vi "Write All Elements Hidden.vi"(8 "error in (no error)":errorcluster, 10 "Config. params. hidden":T1={"Image border size"=1, "Framegrabber board"=0, "Framegrabber buffer"=1, "Camera config file"=path "Support files/camera-config.mcf", "Framegrabber DLL file"=path "C:/CameraVision/Configuration/camera-config.mcf"} {"Framegrabber buffer" min=1; "Framegrabber board" min=0; "Image border size" min=0}, 11 "Config params in":refnum<class "CV-Configuration.lvclass">) -> (0 "error out":errorcluster, 3 "Config params out":refnum<class "CV-Configuration.lvclass">)   [LabVIEW 2013, in "CameraVision.lvlib" / "CV-Configuration.lvclass"]
uses:
  CV-Configuration.lvclass
  Configuration-parameters-advanced.ctl
  CV-Configuration.lvclass/CV-Configuration.ctl
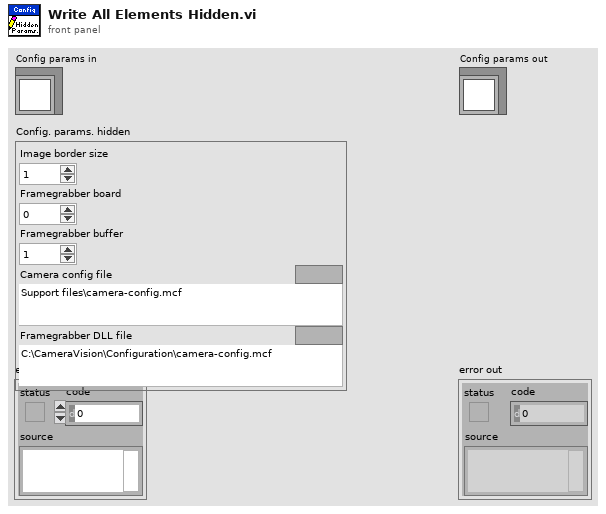
[diagram p1: front panel]
types:
  T1 = typedef "CameraVision.lvlib/CV-Configuration.lvclass/Configuration-parameters-advanced.ctl" = cluster{"Image border size":i32, "Framegrabber board":i32, "Framegrabber buffer":i32, "Camera config file":path, "Framegrabber DLL file":path}
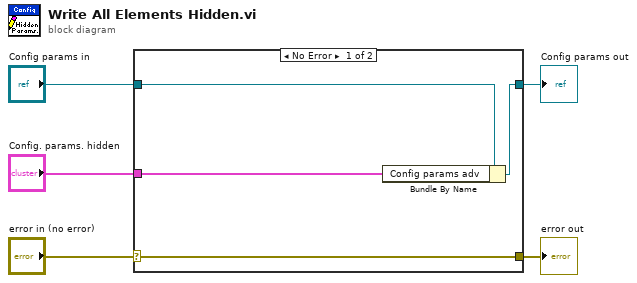
[diagram p0: block diagram]
diagram:
  n1 = case shown="No Error" "error in (no error)" {
    selector: "error in (no error)" -> [w9 w10]
    tunnel: [w9 w10] -> w4
    tunnel: [w7 w11] -> w2
    tunnel: "Config params in" -> [w8 w11]
    tunnel: "Config. params. hidden" -> [w6 _]
    frame No Error {
      n2 = Bundle By Name(cluster=w8, "Config params adv"=w6) -> (w7:refnum<class "CV-Configuration.lvclass">)
    }
    frame Error {
    }
  }
  "error out" <- w4
  "Config params out" <- w2
